vi "Get Server Internal UEs.vi"(11 "OOP Server in":refnum<class "HVC3.lvclass">) -> (2 "Server Internal UEs":T1, 3 "OOP Server out":refnum<class "HVC3.lvclass">)   [LabVIEW 2019, in "HVC3.lvlib" / "HVC3.lvclass"]
uses:
  HVC3.lvclass
  typeDefs/Server Internal UEs.ctl
  typeDefs/Server Internal Message.ctl
  HVC3.lvclass/HVC3.ctl
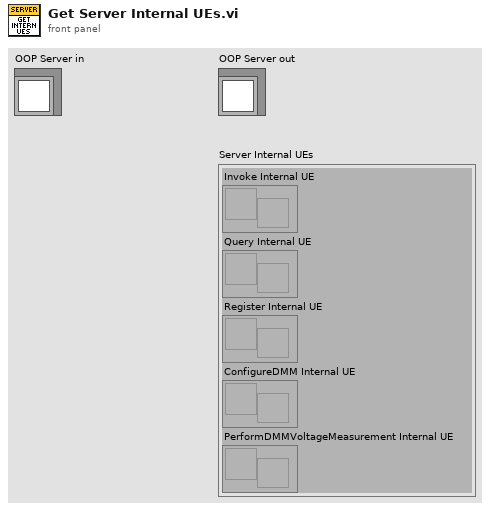
[diagram p1: front panel]
types:
  T1 = typedef "HVC3.lvlib/HVC3.lvclass/Server Internal UEs.ctl" = cluster{"Invoke Internal UE":refnum<user-event>, "Query Internal UE":refnum<user-event>, "Register Internal UE":refnum<user-event>, "ConfigureDMM Internal UE":refnum<user-event>, "PerformDMMVoltageMeasurement Internal UE":refnum<user-event>}
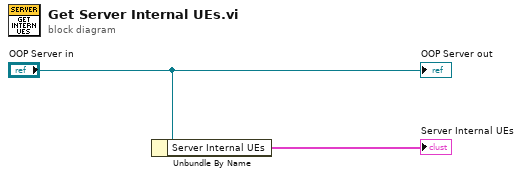
[diagram p0: block diagram]
diagram:
  n1 = Unbundle By Name("OOP Server in") -> ("Server Internal UEs"=→"Server Internal UEs":T1)
  "OOP Server out" <- "OOP Server in"
